vi "MainTester.vi"() -> ()   [LabVIEW 2015]
uses:
  <vilib>/Rock Robotics/WPI/SerialPort/WPI_SerialPortRef.ctl
panel:
  in  "stop":bool
  out "error out":errorcluster
  out "SerialPortRef 2":T1
  out "32 bit array":bool[](array[boolean])
  in  "error in (no error)":errorcluster
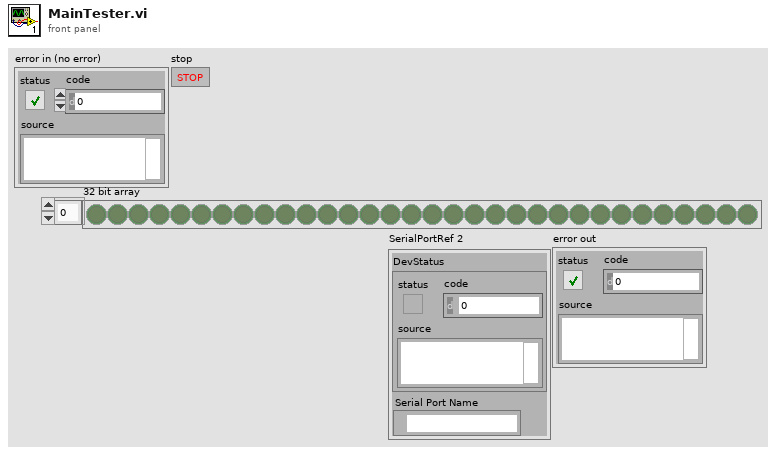
[diagram p1: front panel]
types:
  T1 = typedef "WPI_SerialPortRef.ctl" = cluster{"DevStatus":errorcluster, "Serial Port Name":refnum<visa-resource-name>}
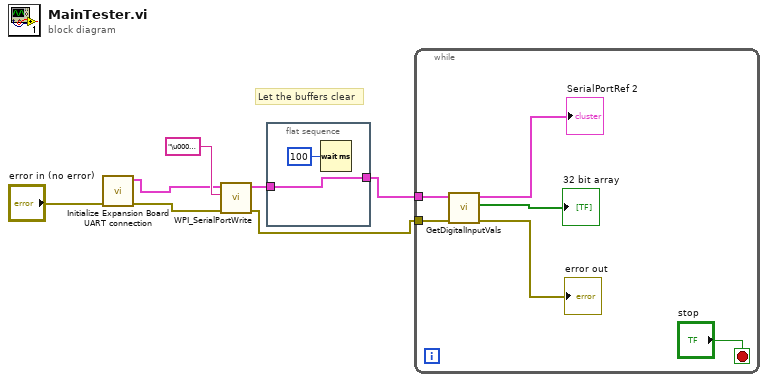
[diagram p0: block diagram]
diagram:
  # "Let the buffers clear"
  n1 = call "Initialize Expansion Board UART connection.vi"("error in (no error)"="error in (no error)") -> ("error out"=w4:errorcluster, "SerialPortRef"=w5:T1)  [unwired: 9 in]
  n2 = call <vilib>:"WPI_SerialPortWrite.vi"("error in (no error)"=w4, "Buffer"="\u0004\u0004", "SerialPortRef"=w5) -> ("error out"=w2:errorcluster, "SerialPortRef"=w3:T1)  [unwired: 6 in, 1 out]
  n3 = flat-sequence {
    tunnel: [w9] -> w1
    tunnel: w3 -> [w9]
    frame #0 {
      n4 = Wait (ms)(milliseconds to wait=u32 100) -> ()  [unwired: 1 out]
    }
  }
  n5 = while {
    tunnel: w2 -> [w15]
    tunnel: w1 -> [w14]
    stop <- "stop" stop-if-true
    n6 = call "GetDigitalInputVals.vi"("error in (no error)"=w15, "SerialPortRef"=w14) -> ("error out"=→"error out":errorcluster, "32 bit array"=→"32 bit array":bool[], "SerialPortRef 2"=→"SerialPortRef 2":T1)  [unwired: 7 in]
  }
